vi "PPMS_Femto_TXT_Global_READ.vi"(3 "Property":u16(ring)=6 items=["1 - DDPCA Gain (V/A)", "2 - DDPCA Gain (V/A)", "3 - DLPVA Gain (dB)", "3 - Gain 1", "3 - Gain 2", "3 - AC/DC coupling", "3 - filter", "4 - DLPVA Gain (dB)", "4 - Gain 1", "4 - Gain 2", "4 - AC/DC coupling", "4 - filter"]) -> (0 "Value":i32=20, 1 "Property":string="4 - DLPVA Gain (dB)")   [LabVIEW 2010]
uses:
  <vilib>/Utility/file.llb/Read From Spreadsheet File (string).vi
panel:
  in  "file path (dialog if empty)":path=path "D:/Labview/PPMS_Femto_TXT_Global.vi.txt"
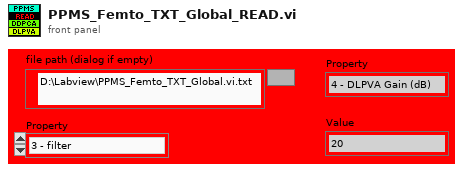
[diagram p1: front panel]
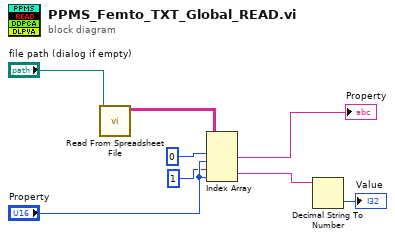
[diagram p0: block diagram]
diagram:
  n1 = call-poly <vilib>:"Read From Spreadsheet File.vi"("file path (dialog if empty)"="file path (dialog if empty)") -> ("all rows"=w7:string[][])  [unwired: 6 in, 4 out]
  n2 = Index Array(array=w7, index (row) #1=0 ("index (row)"), index (col) #1="Property", index (row) #2=1 ("disabled index (row)"), index (col) #2="Property") -> (element #1=→"Property":string, element #2=w1:string)
  n3 = Decimal String To Number(string=w1) -> (number=→"Value":i32)  [unwired: 2 in, 1 out]
